vi "SpeedCache.vi"(6 "size of this data block":dbl=1.0, 7 "operation":T1, 8 "error in (no error)":errorcluster, 9 "pulse position data":dbl[](array[numeric]), 10 "max empty blocks":i32, 11 "channel":string) -> (0 "error out":errorcluster, 2 "speed (RPM)":dbl, 3 "pulse cache":T2)   [LabVIEW 2017, in "AnalysisHelper.lvlib"]
uses:
  <vilib>/addons/InsightCM/Utilities/Analysis/Shared/AnalysisHelper.lvlib
  <vilib>/addons/InsightCM/Utilities/Analysis/Shared/controls/SpeedCache.ctl
  <vilib>/addons/InsightCM/Utilities/Analysis/Shared/controls/SpeedCacheOps.ctl
panel:
  out "empty blocks":i32
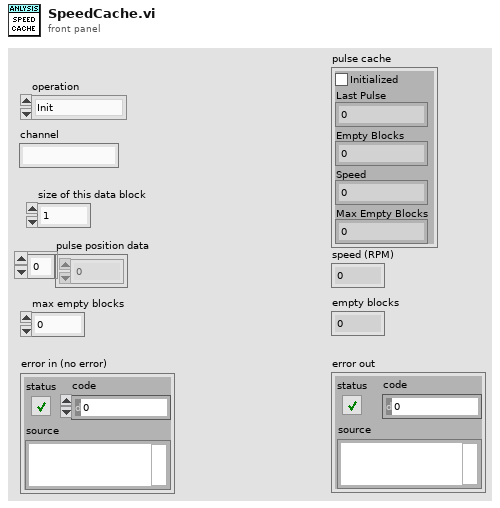
[diagram p1: front panel]
types:
  T1 = typedef "AnalysisHelper.lvlib/SpeedCacheOps.ctl" = enum16{"Init", "GetSpeed"}
  T2 = typedef "AnalysisHelper.lvlib/SpeedCache.ctl" = cluster{"Initialized":bool, "Last Pulse":dbl, "Empty Blocks":i32, "Speed":dbl, "Max Empty Blocks":i32}
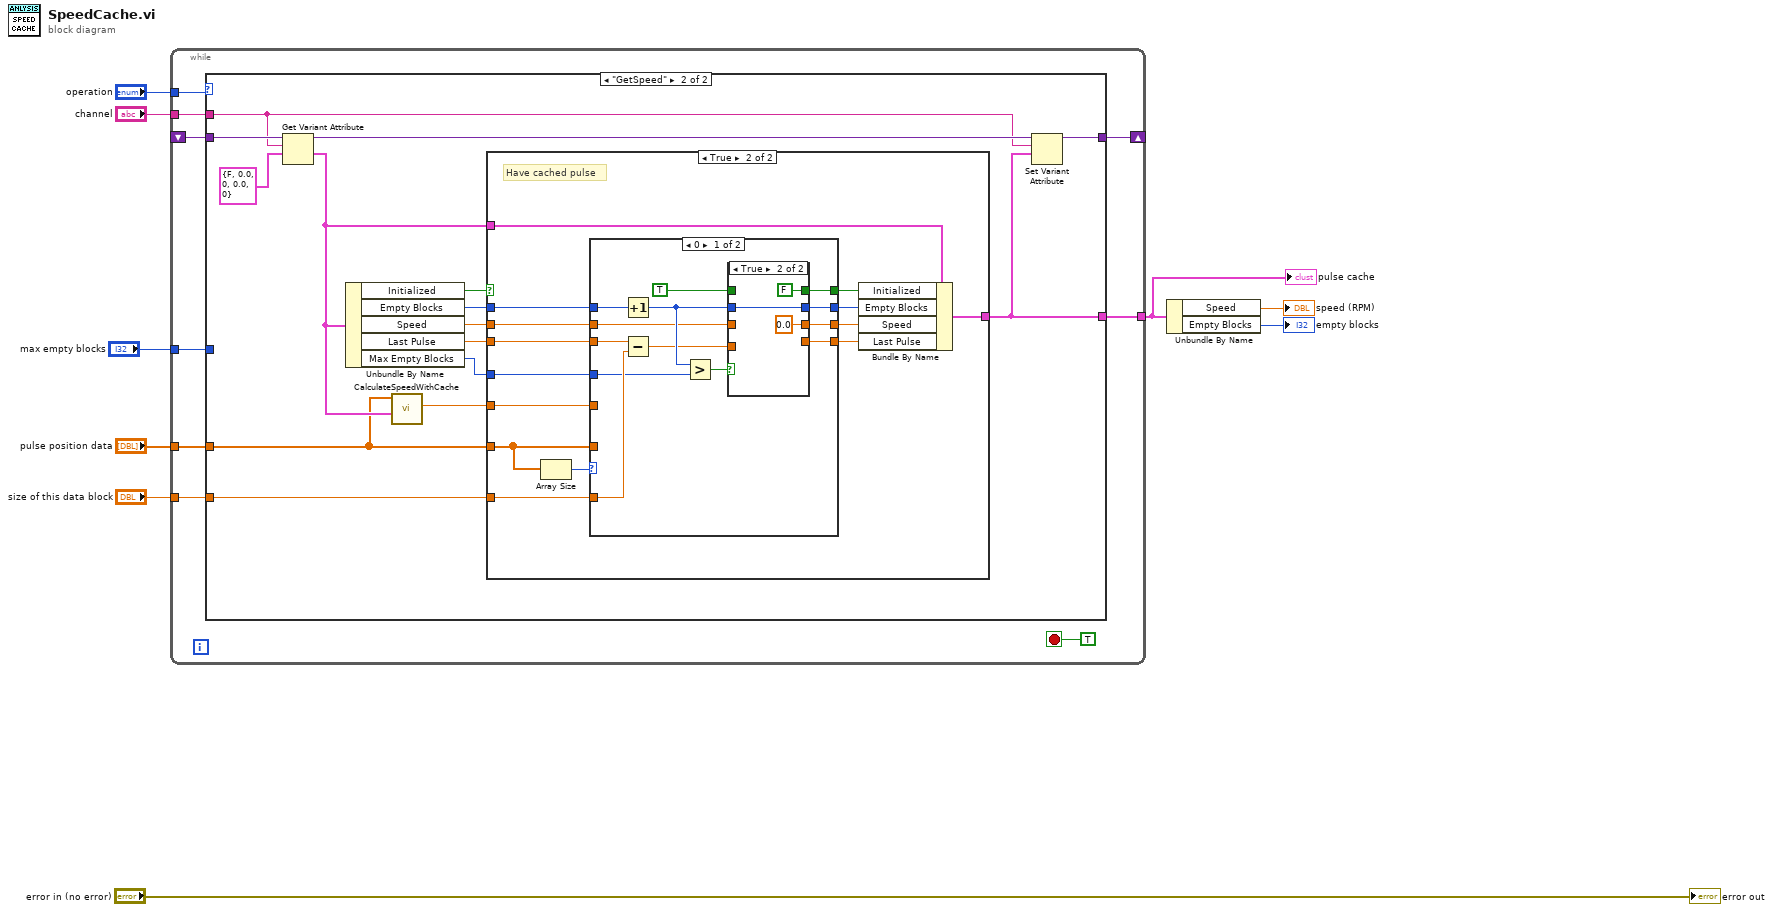
[diagram p0: block diagram]
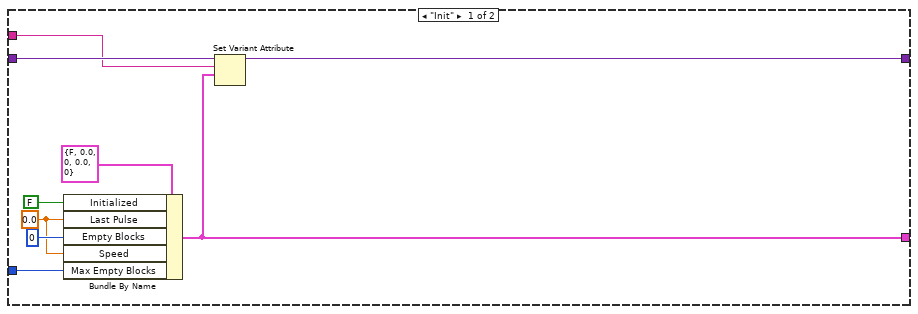
[diagram p2: hidden frame]
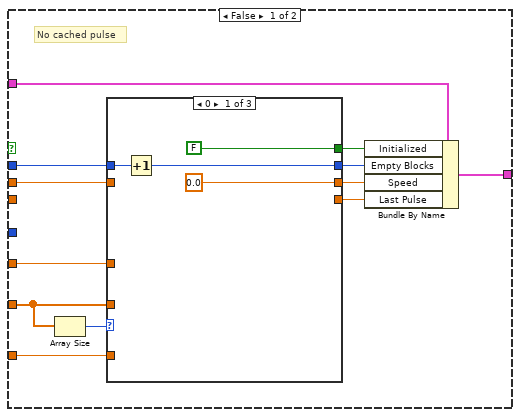
[diagram p3: hidden frame]
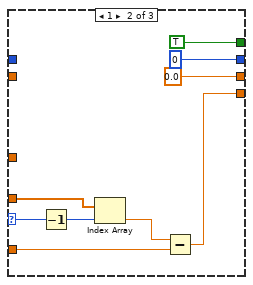
[diagram p4: hidden frame]
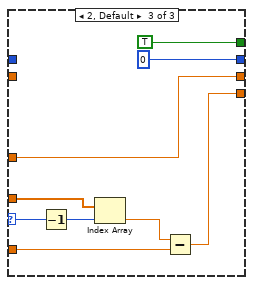
[diagram p5: hidden frame]
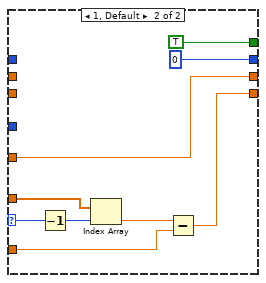
[diagram p7: hidden frame]
diagram:
  n1 = while {
    tunnel: "channel" -> [w17]
    shift-right: [w16] -> _
    shift-left: _ -> [w15]
    tunnel: "pulse position data" -> [w14]
    tunnel: "size of this data block" -> [w13]
    tunnel: [w12] -> w6
    tunnel: "operation" -> [w11]
    tunnel: "max empty blocks" -> [w10]
    stop <- TRUE stop-if-true
    n2 = case shown="\"GetSpeed\"" w11 {
      tunnel: w17 -> [w26 w37]
      tunnel: [w25 w38] -> w16
      tunnel: w15 -> [w27 w42]
      tunnel: w14 -> [_ w32]
      tunnel: w13 -> [_ w35]
      tunnel: [w19 w36] -> w12
      tunnel: w10 -> [w20 _]
      frame "Init" {
        w21 = 0.0 ("Last Pulse")
        n3 = Bundle By Name(cluster=T2 {"Initialized"=FALSE, "Last Pulse"=0.0, "Empty Blocks"=0, "Speed"=0.0, "Max Empty Blocks"=0} ("DataStoreType"), "Initialized"=FALSE, "Last Pulse"=w21, "Empty Blocks"=0, "Speed"=w21, "Max Empty Blocks"=w20) -> (w19:T2)
        n4 = Set Variant Attribute(Variant=w27, name=w26, value=w19) -> (Variant out=w25:variant)  [unwired: 1 in, 2 out]
      }
      frame "GetSpeed" {
        n5 = Get Variant Attribute(Variant=w42, name=w37, default value (empty Variant)=T2 {"Initialized"=FALSE, "Last Pulse"=0.0, "Empty Blocks"=0, "Speed"=0.0, "Max Empty Blocks"=0} ("Pulse Cache Type")) -> (duplicate Variant=w39:variant, value=w33:T2)  [unwired: 1 in, 2 out]
        n6 = Unbundle By Name(w33) -> ("Initialized"=w34:bool, "Empty Blocks"=w40:i32, "Speed"=w30:dbl, "Last Pulse"=w31:dbl, "Max Empty Blocks"=w28:i32)
        n7 = call <vilib>:"CalculateSpeedWithCache.vi"("pulse cache"=w33, "Pulse Positions"=w32) -> ("Speed (RPM)"=w29:dbl)  [unwired: 8 in, 1 out]
        n8 = case shown="True" w34 {
          tunnel: w32 -> [w49 w84]
          tunnel: w33 -> [w54 w82]
          tunnel: w40 -> [w52 w88]
          tunnel: w31 -> [_ w83]
          tunnel: [w51 w87] -> w36
          tunnel: w35 -> [w50 w86]
          tunnel: w30 -> [w45 w79]
          tunnel: w29 -> [w43 w78]
          tunnel: w28 -> [_ w77]
          frame False {
            # "No cached pulse"
            n9 = Array Size(array=w49) -> (size(s)=w53:i32)
            n10 = case shown="0" w53 {
              selector: w53 -> [_ w66 w75]
              tunnel: w52 -> [w58 _ _]
              tunnel: w49 -> [_ w67 w76]
              tunnel: w50 -> [_ w64 w73]
              tunnel: [FALSE ("Initialized") TRUE ("Initialized") TRUE ("Initialized")] -> w48
              tunnel: [w57 0 0] -> w47
              tunnel: [_ w60 w69] -> w46
              tunnel: w45 -> [_ _ _]
              tunnel: [0.0 0.0 w68] -> w44
              tunnel: w43 -> [_ _ w68]
              frame 0 {
                n11 = Increment(x=w58) -> (x+1=w57:i32)
              }
              frame 1 {
                n12 = Decrement(x=w66) -> (x-1=w65:i32)
                n13 = Index Array(array=w67, index=w65) -> (element=w63:dbl)
                n14 = Subtract(x=w63, y=w64) -> (x-y=w60:dbl)
              }
              frame 2, Default {
                n15 = Decrement(x=w75) -> (x-1=w74:i32)
                n16 = Index Array(array=w76, index=w74) -> (element=w72:dbl)
                n17 = Subtract(x=w72, y=w73) -> (x-y=w69:dbl)
              }
            }
            n18 = Bundle By Name(cluster=w54, "Initialized"=w48, "Empty Blocks"=w47, "Speed"=w44, "Last Pulse"=w46) -> (w51:T2)
          }
          frame True {
            # "Have cached pulse"
            n19 = Array Size(array=w84) -> (size(s)=w90:i32)
            n20 = case shown="0" w90 {
              selector: w90 -> [_ w118]
              tunnel: [w96 0] -> w89
              tunnel: w88 -> [w103 _]
              tunnel: [w98 TRUE ("Initialized")] -> w85
              tunnel: [w92 w114] -> w81
              tunnel: w84 -> [_ w116]
              tunnel: w83 -> [w102 _]
              tunnel: w86 -> [w101 w112]
              tunnel: [w94 w111] -> w80
              tunnel: w79 -> [w93 _]
              tunnel: w78 -> [_ w111]
              tunnel: w77 -> [w100 _]
              frame 0 {
                n21 = Increment(x=w103) -> (x+1=w95:i32)
                n22 = Subtract(x=w102, y=w101) -> (x-y=w91:dbl)
                n23 = Greater?(x=w95, y=w100) -> (0:w99:bool)
                n24 = case shown="True" w99 {
                  tunnel: [w107 FALSE ("Initialized")] -> w98
                  tunnel: TRUE ("Initialized") -> [w107 _]
                  tunnel: [w106 w109] -> w96
                  tunnel: w95 -> [w106 w109]
                  tunnel: [w105 0.0 ("Speed")] -> w94
                  tunnel: w93 -> [w105 _]
                  tunnel: [w104 _] -> w92
                  tunnel: w91 -> [w104 _]
                  frame False {
                  }
                  frame True {
                  }
                }
              }
              frame 1, Default {
                n25 = Decrement(x=w118) -> (x-1=w117:i32)
                n26 = Index Array(array=w116, index=w117) -> (element=w115:dbl)
                n27 = Subtract(x=w115, y=w112) -> (x-y=w114:dbl)
              }
            }
            n28 = Bundle By Name(cluster=w82, "Initialized"=w85, "Empty Blocks"=w89, "Speed"=w80, "Last Pulse"=w81) -> (w87:T2)
          }
        }
        n29 = Set Variant Attribute(Variant=w39, name=w37, value=w36) -> (Variant out=w38:variant)  [unwired: 1 in, 2 out]
      }
    }
  }
  "pulse cache" <- w6
  n30 = Unbundle By Name(w6) -> ("Speed"=→"speed (RPM)":dbl, "Empty Blocks"=→"empty blocks":i32)
  "error out" <- "error in (no error)"
